vi "Channels to Define.vi"(8 "error in (no error)":errorcluster, 11 "Abstract Routing Channel Template in":refnum<class "Abstract Routing Channel Template.lvclass">) -> (0 "error out":errorcluster, 2 "Channels":string[](array[string]), 3 "Abstract Routing Channel Template out":refnum<class "Abstract Routing Channel Template.lvclass">)   [LabVIEW 2020, in "Routing Templates.lvlib" / "Abstract Routing Channel Template.lvclass"]
uses:
  Abstract Routing Channel Template.lvclass
  Abstract Routing Channel Template.lvclass/Abstract Routing Channel Template.ctl
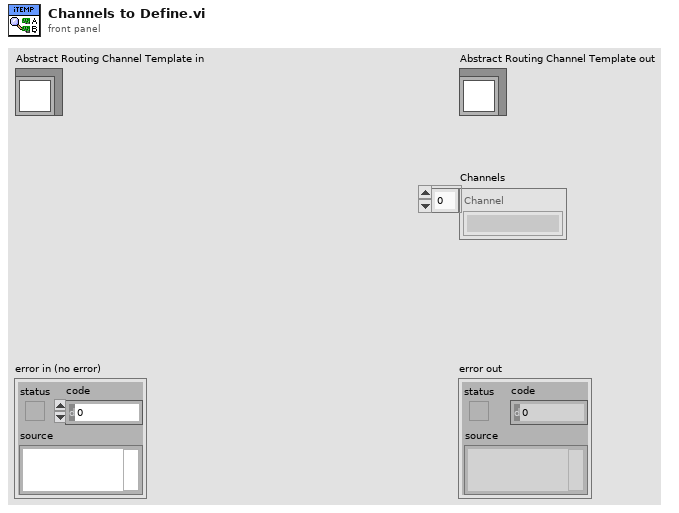
[diagram p1: front panel]
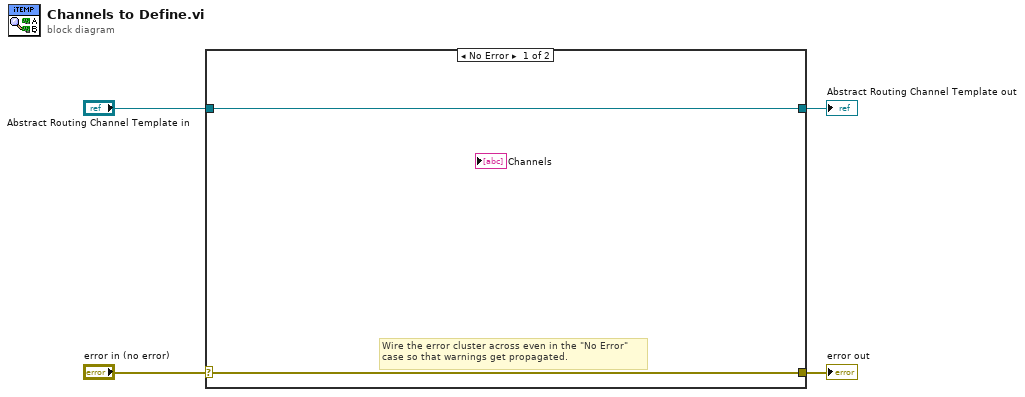
[diagram p0: block diagram]
diagram:
  n1 = case shown="No Error" "error in (no error)" {
    selector: "error in (no error)" -> [w5 w8]
    tunnel: [w5 w8] -> w3
    tunnel: [w6 w7] -> w1
    tunnel: "Abstract Routing Channel Template in" -> [w6 w7]
    frame No Error {
      # "Wire the error cluster across even in the \"No Error\"\ncase so that warnings get propagated."
    }
    frame Error {
    }
  }
  "error out" <- w3
  "Abstract Routing Channel Template out" <- w1
